vi "Timed Message_Start.vi"(0 "Message":string, 5 "Address":string, 7 "Interval":i32=1000 format="%dmsec", 9 "Timeout":i32=1000 format="%dmsec", 11 "error in":errorcluster) -> (4 "FTW Actor Connector":refnum<class "Timed Message.lvclass">, 6 "Initialized Response":string, 8 "Instance Inbox Address":string, 10 "Instance Publisher Address":string, 15 "error out":errorcluster)   [LabVIEW 2012, in "Timed Message.lvclass"]
uses:
  Timed Message.lvclass
  src/Connector/FTW-ActorConnector.lvclass
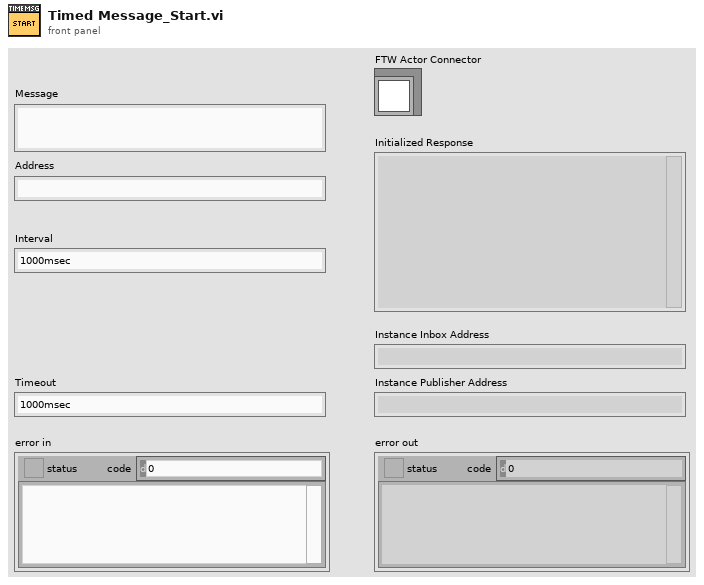
[diagram p1: front panel]
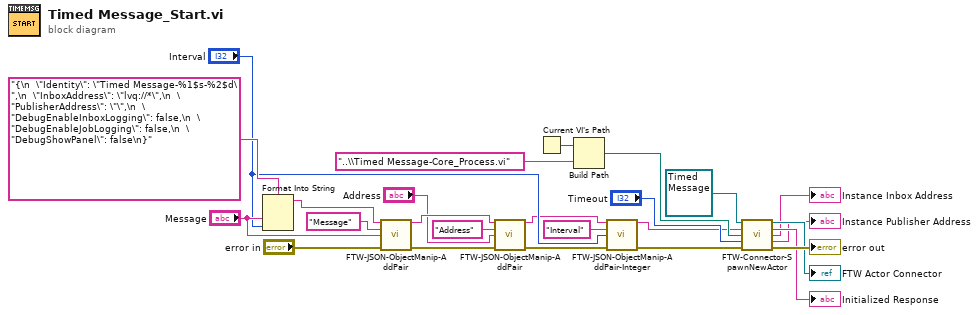
[diagram p0: block diagram]
diagram:
  n1 = Format Into String(format string="{\n  \"Identity\": \"Timed Message-%1$s-%2$d\",\n  \"InboxAddress\": \"lvq://*\",\n  \"PublisherAddress\": \"\",\n  \"DebugEnableInboxLogging\": false,\n  \"DebugEnableJobLogging\": false,\n  \"DebugShowPanel\": false\n}" ("Configuration"), "Message", "Interval") -> (resulting string=w8:string)  [unwired: 2 in, 1 out]
  n2 = call "FTW-JSON-ObjectManip-AddPair.vi"("Input JSON Object"=w8, "Key"="Message", "Value"="Message", "error in"="error in") -> ("Output JSON Object"=w4:string, "error out"=w14:errorcluster)  [unwired: 10 in]
  n3 = call "FTW-JSON-ObjectManip-AddPair.vi"("Input JSON Object"=w4, "Key"="Address", "Value"="Address", "error in"=w14) -> ("Output JSON Object"=w3:string, "error out"=w5:errorcluster)  [unwired: 10 in]
  n4 = Current VI's Path() -> (path=w23:path)
  n5 = Build Path(base path=w23, name or relative path="..\\Timed Message-Core_Process.vi") -> (appended path=w21:path)
  n6 = call "FTW-JSON-ObjectManip-AddPair-Integer.vi"("Input JSON Object"=w3, "Key"="Interval", "Value"="Interval", "error in"=w5) -> ("Output JSON Object"=w12:string, "error out"=w13:errorcluster)  [unwired: 10 in]
  n7 = call "FTW-Connector-SpawnNewActor.vi"("FTW Actor Connector Type"=refnum<class "Timed Message.lvclass"> refnum ("TTK_Splashscreen.lvclass"), "Configuration"=w12, "Actor VI Filepath"=w21, "Timeout"="Timeout", "error in"=w13) -> ("FTW Actor Connector"=→"FTW Actor Connector":refnum<class "Timed Message.lvclass">, "Initialized Response"=→"Initialized Response":string, "Instance Inbox Address"=→"Instance Inbox Address":string, "Instance Publisher Address"=→"Instance Publisher Address":string, "error out"=→"error out":errorcluster)  [unwired: 6 in]
